vi "Process Array Elements.vi"(7 "Format String (%#0.15f)":string="%#0.15f", 8 "Error In":errorcluster, 9 "Name In":string, 10 "Array Variant":variant, 11 "Queue In":refnum<queue>) -> (0 "Error Out":errorcluster, 1 "Data Out":string, 3 "Queue Out":refnum<queue>)   [LabVIEW 2020]
doc: "This VI was created for use with the Read/Write Cluster VIs. It converts array elements of the cluster to strings to be written to file.\n\nFreeware from Moore Good Ideas, www.mooregoodideas.com. Do not remove this line."
uses:
  <vilib>/Utility/Data Type/NI_Data Type.lvlib
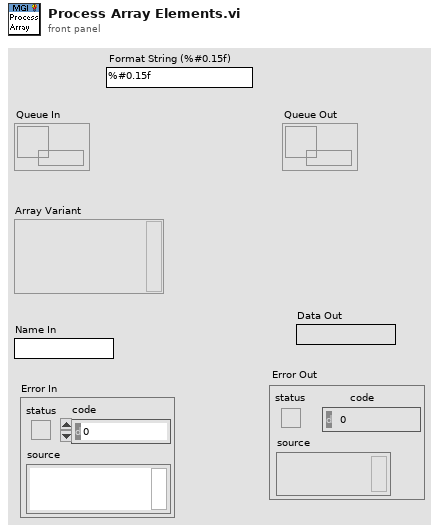
[diagram p1: front panel]
types:
  T1 = typedef "NI_Data Type.lvlib/Data Type.ctl" = enum8{"Invalid Type", "Void", "I8", "I16", "I32", "I64", "U8", "U16", "U32", "U64", "Single Float", "Double Float", "Extended Float", "Single Complex", "Double Complex", "Extended Complex", "Enum U8", "Enum U16", "Enum U32", "Enum U64", "Single Float With Unit", "Double Float With Unit", "Extended Float With Unit", "Single Complex with Unit", "Double Complex with Unit", "Extended Complex with Unit", "Boolean", "String", "Path", "Picture", "Tag", "Array", "Cluster", "Variant", "LV Variant", "Waveform", "Timestamp", "Digital Waveform", "Digital Data", "ExpressData", "Refnum", "External Data", "VI", "Poly VI", "LabVIEW Class Instance", "Fixed Point", "Set Collection", "Map Collection"}
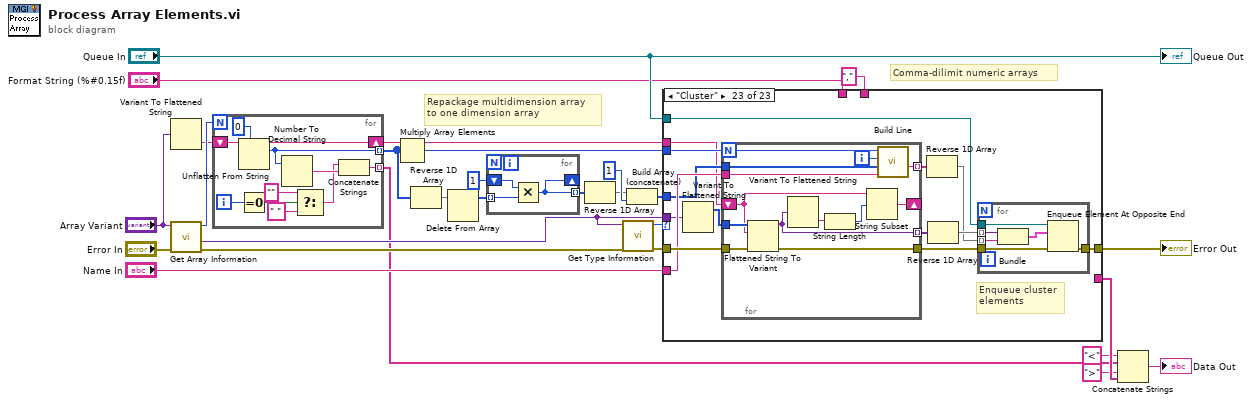
[diagram p0: block diagram]
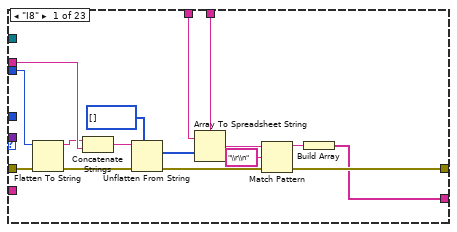
[diagram p2: hidden frame]
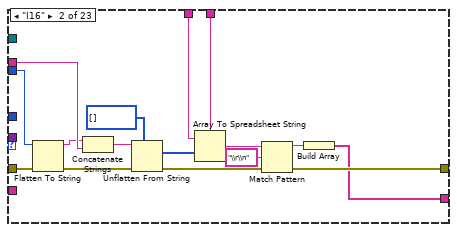
[diagram p3: hidden frame]
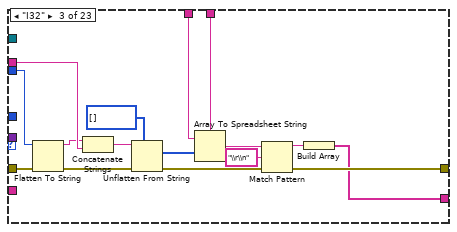
[diagram p4: hidden frame]
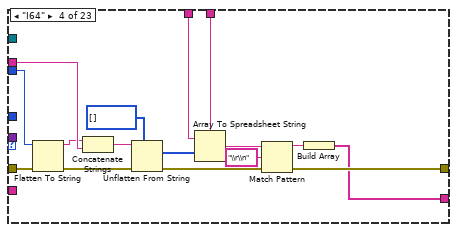
[diagram p5: hidden frame]
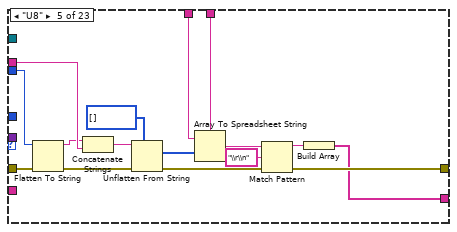
[diagram p6: hidden frame]
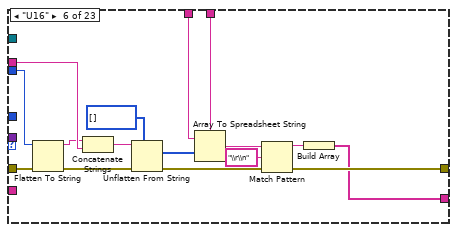
[diagram p7: hidden frame]
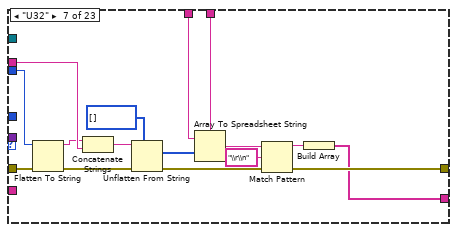
[diagram p8: hidden frame]
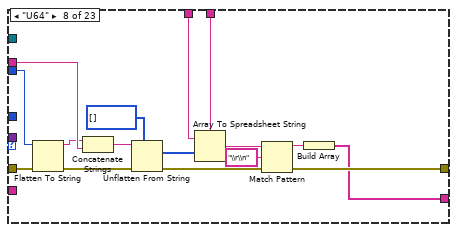
[diagram p9: hidden frame]
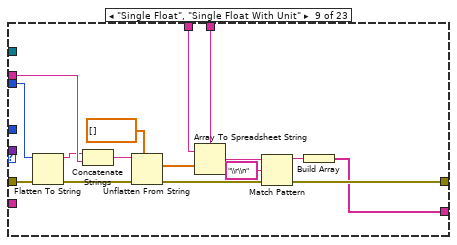
[diagram p10: hidden frame]
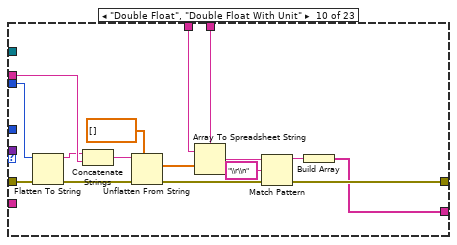
[diagram p11: hidden frame]
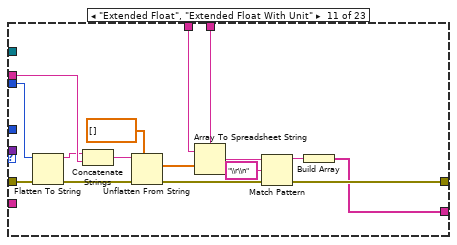
[diagram p12: hidden frame]
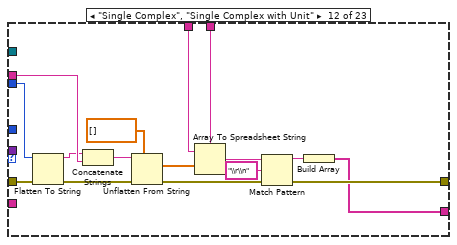
[diagram p13: hidden frame]
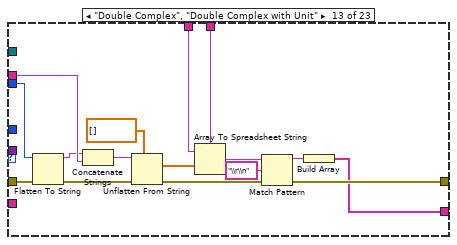
[diagram p14: hidden frame]
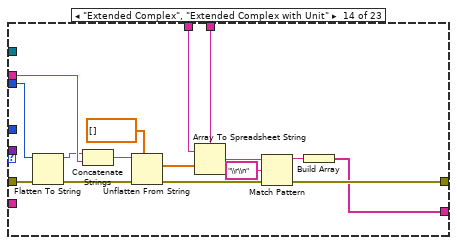
[diagram p15: hidden frame]
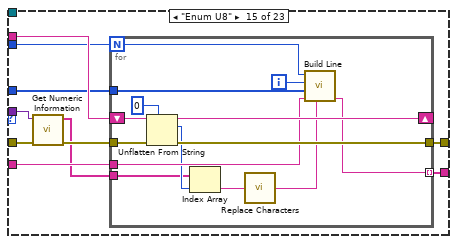
[diagram p16: hidden frame]
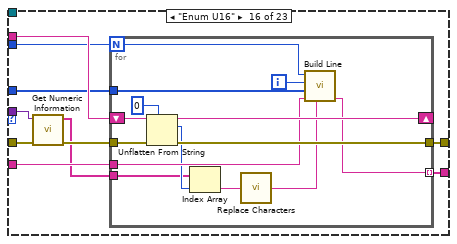
[diagram p17: hidden frame]
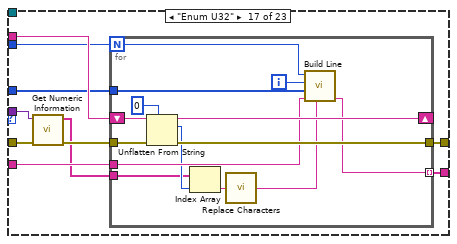
[diagram p18: hidden frame]
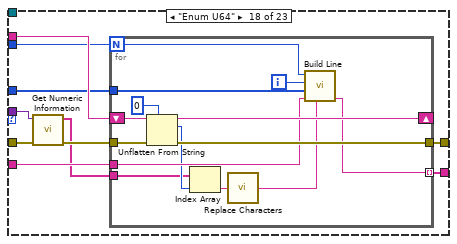
[diagram p19: hidden frame]
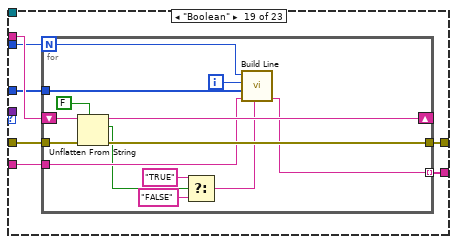
[diagram p20: hidden frame]
diagram:
  # "Comma-dilimit numeric arrays"
  # "Repackage multidimension array\nto one dimension array"
  n1 = Variant To Flattened String(Variant="Array Variant") -> (data string=w25:string)  [unwired: 1 out]
  n2 = call <vilib>:"Get Array Information.vi"("error in (no error)"="Error In", "variant"="Array Variant") -> ("error out"=w7:errorcluster, "array element data type"=w8:variant, "number of dimensions"=w26:i32)  [unwired: 6 in, 1 out]
  n3 = for {
    N: w26 -> [_]
    shift-right: [w37] -> w23
    shift-left: w25 -> [w38]
    tunnel: [w34] -> w12 mode=indexing
    tunnel: [w35] -> w6 mode=indexing
    i -> [w33]
    n4 = Unflatten From String(type=u32 0, binary string=w38) -> (rest of the binary string=w37:string, value=w34:u32)  [unwired: 3 in, 1 out]
    n5 = Equal To 0?(x=w33) -> (x = 0?=w32:bool)
    n6 = Number To Decimal String(number=w34) -> (decimal integer string=w36:string)  [unwired: 1 in]
    n7 = Select(t="", s=w32, f=" ") -> (s? t:f=w30:string)
    n8 = Concatenate Strings(w30, w36) -> (w35:string)
  }
  n9 = Multiply Array Elements(1:w12) -> (0:w22:u32)
  n10 = Reverse 1D Array(array=w12) -> (reversed array=w13:u32[])
  n11 = Delete From Array(array=w13) -> (array with subset deleted=w14:u32[])  [unwired: 2 in, 1 out]
  n12 = for {
    tunnel: w14 -> [w42] mode=indexing
    shift-right: [w40] -> _
    shift-left: i8 1 -> [w41]
    tunnel: [w40] -> w16 mode=indexing
    n13 = Multiply(x=w41, y=w42) -> (x*y=w40:u32)
  }
  n14 = Reverse 1D Array(array=w16) -> (reversed array=w17:u32[])
  n15 = call <vilib>:"Get Type Information.vi"("error in (no error)"=w7, "variant"=w8) -> ("error out"=w24:errorcluster, "type"=w3:T1)  [unwired: 5 in, 3 out]
  n16 = Build Array (concatenate)(w17, i8 1) -> (w11:u32[])
  n17 = case shown="\"Cluster\"" w3 {
    tunnel: [w57 w72 w87 w102 w117 w132 w147 w162 w177 w192 w207 w222 w237 w252 w262 w286 w310 w334 w355 w376 w395 w411 w421] -> w10
    tunnel: w24 -> [w46 w61 w76 w91 w106 w121 w136 w151 w166 w181 w196 w211 w226 w241 w255 w279 w303 w327 w354 w375 w394 w411 w429]
    tunnel: w23 -> [w56 w71 w86 w101 w116 w131 w146 w161 w176 w191 w206 w221 w236 w251 w261 w285 w309 w333 w353 w374 w393 w410 w416]
    tunnel: w22 -> [w55 w70 w85 w100 w115 w130 w145 w160 w175 w190 w205 w220 w235 w250 w260 w284 w308 w332 w352 w373 w392 _ w428]
    tunnel: "Name In" -> [_ _ _ _ _ _ _ _ _ _ _ _ _ _ w259 w283 w307 w331 w351 w372 w391 _ w427]
    tunnel: [w54 w69 w84 w99 w114 w129 w144 w159 w174 w189 w204 w219 w234 w249 w257 w281 w305 w329 w349 w370 w389 w409 _] -> w20
    tunnel: w11 -> [_ _ _ _ _ _ _ _ _ _ _ _ _ _ w258 w282 w306 w330 w350 w371 w390 _ w426]
    tunnel: "Queue In" -> [_ _ _ _ _ _ _ _ _ _ _ _ _ _ _ _ _ _ _ _ _ _ w422]
    tunnel: w8 -> [_ _ _ _ _ _ _ _ _ _ _ _ _ _ w256 w280 w304 w328 _ _ _ _ w419]
    tunnel: "Format String (%#0.15f)" -> [w44 w59 w74 w89 w104 w119 w134 w149 w164 w179 w194 w209 w224 w239 _ _ _ _ _ _ _ _ _]
    tunnel: "," ("delimiter (Tab)") -> [w43 w58 w73 w88 w103 w118 w133 w148 w163 w178 w193 w208 w223 w238 _ _ _ _ _ _ _ _ _]
    frame "I8" {
      n18 = Flatten To String(anything=w55, error in (no error)=w46) -> (data string=w51:string, error out=w45:errorcluster)  [unwired: 2 in, 1 out]
      n19 = Concatenate Strings(w51, w56) -> (w52:string)
      n20 = Unflatten From String(type=i8[] [], binary string=w52, error in (no error)=w45) -> (value=w48:i8[], error out=w57:errorcluster)  [unwired: 2 in, 1 out]
      n21 = Array To Spreadsheet String(delimiter (Tab)=w43, array=w48, 3:w44) -> (spreadsheet string=w50:string)
      n22 = Match Pattern(string=w50, regular expression="\\r\\n") -> (before substring=w47:string)  [unwired: 1 in, 3 out]
      n23 = Build Array(w47) -> (w54:string[])
    }
    frame "I16" {
      n24 = Flatten To String(anything=w70, error in (no error)=w61) -> (data string=w66:string, error out=w60:errorcluster)  [unwired: 2 in, 1 out]
      n25 = Concatenate Strings(w66, w71) -> (w67:string)
      n26 = Unflatten From String(type=i16[] [], binary string=w67, error in (no error)=w60) -> (value=w63:i16[], error out=w72:errorcluster)  [unwired: 2 in, 1 out]
      n27 = Array To Spreadsheet String(delimiter (Tab)=w58, array=w63, 3:w59) -> (spreadsheet string=w65:string)
      n28 = Match Pattern(string=w65, regular expression="\\r\\n") -> (before substring=w62:string)  [unwired: 1 in, 3 out]
      n29 = Build Array(w62) -> (w69:string[])
    }
    frame "I32" {
      n30 = Flatten To String(anything=w85, error in (no error)=w76) -> (data string=w81:string, error out=w75:errorcluster)  [unwired: 2 in, 1 out]
      n31 = Concatenate Strings(w81, w86) -> (w82:string)
      n32 = Unflatten From String(type=i32[] [], binary string=w82, error in (no error)=w75) -> (value=w78:i32[], error out=w87:errorcluster)  [unwired: 2 in, 1 out]
      n33 = Array To Spreadsheet String(delimiter (Tab)=w73, array=w78, 3:w74) -> (spreadsheet string=w80:string)
      n34 = Match Pattern(string=w80, regular expression="\\r\\n") -> (before substring=w77:string)  [unwired: 1 in, 3 out]
      n35 = Build Array(w77) -> (w84:string[])
    }
    frame "I64" {
      n36 = Flatten To String(anything=w100, error in (no error)=w91) -> (data string=w96:string, error out=w90:errorcluster)  [unwired: 2 in, 1 out]
      n37 = Concatenate Strings(w96, w101) -> (w97:string)
      n38 = Unflatten From String(type=i64[] [], binary string=w97, error in (no error)=w90) -> (value=w93:i64[], error out=w102:errorcluster)  [unwired: 2 in, 1 out]
      n39 = Array To Spreadsheet String(delimiter (Tab)=w88, array=w93, 3:w89) -> (spreadsheet string=w95:string)
      n40 = Match Pattern(string=w95, regular expression="\\r\\n") -> (before substring=w92:string)  [unwired: 1 in, 3 out]
      n41 = Build Array(w92) -> (w99:string[])
    }
    frame "U8" {
      n42 = Flatten To String(anything=w115, error in (no error)=w106) -> (data string=w111:string, error out=w105:errorcluster)  [unwired: 2 in, 1 out]
      n43 = Concatenate Strings(w111, w116) -> (w112:string)
      n44 = Unflatten From String(type=u8[] [], binary string=w112, error in (no error)=w105) -> (value=w108:u8[], error out=w117:errorcluster)  [unwired: 2 in, 1 out]
      n45 = Array To Spreadsheet String(delimiter (Tab)=w103, array=w108, 3:w104) -> (spreadsheet string=w110:string)
      n46 = Match Pattern(string=w110, regular expression="\\r\\n") -> (before substring=w107:string)  [unwired: 1 in, 3 out]
      n47 = Build Array(w107) -> (w114:string[])
    }
    frame "U16" {
      n48 = Flatten To String(anything=w130, error in (no error)=w121) -> (data string=w126:string, error out=w120:errorcluster)  [unwired: 2 in, 1 out]
      n49 = Concatenate Strings(w126, w131) -> (w127:string)
      n50 = Unflatten From String(type=u16[] [], binary string=w127, error in (no error)=w120) -> (value=w123:u16[], error out=w132:errorcluster)  [unwired: 2 in, 1 out]
      n51 = Array To Spreadsheet String(delimiter (Tab)=w118, array=w123, 3:w119) -> (spreadsheet string=w125:string)
      n52 = Match Pattern(string=w125, regular expression="\\r\\n") -> (before substring=w122:string)  [unwired: 1 in, 3 out]
      n53 = Build Array(w122) -> (w129:string[])
    }
    frame "U32" {
      n54 = Flatten To String(anything=w145, error in (no error)=w136) -> (data string=w141:string, error out=w135:errorcluster)  [unwired: 2 in, 1 out]
      n55 = Concatenate Strings(w141, w146) -> (w142:string)
      n56 = Unflatten From String(type=u32[] [], binary string=w142, error in (no error)=w135) -> (value=w138:u32[], error out=w147:errorcluster)  [unwired: 2 in, 1 out]
      n57 = Array To Spreadsheet String(delimiter (Tab)=w133, array=w138, 3:w134) -> (spreadsheet string=w140:string)
      n58 = Match Pattern(string=w140, regular expression="\\r\\n") -> (before substring=w137:string)  [unwired: 1 in, 3 out]
      n59 = Build Array(w137) -> (w144:string[])
    }
    frame "U64" {
      n60 = Flatten To String(anything=w160, error in (no error)=w151) -> (data string=w156:string, error out=w150:errorcluster)  [unwired: 2 in, 1 out]
      n61 = Concatenate Strings(w156, w161) -> (w157:string)
      n62 = Unflatten From String(type=u64[] [], binary string=w157, error in (no error)=w150) -> (value=w153:u64[], error out=w162:errorcluster)  [unwired: 2 in, 1 out]
      n63 = Array To Spreadsheet String(delimiter (Tab)=w148, array=w153, 3:w149) -> (spreadsheet string=w155:string)
      n64 = Match Pattern(string=w155, regular expression="\\r\\n") -> (before substring=w152:string)  [unwired: 1 in, 3 out]
      n65 = Build Array(w152) -> (w159:string[])
    }
    frame "Single Float", "Single Float With Unit" {
      n66 = Flatten To String(anything=w175, error in (no error)=w166) -> (data string=w171:string, error out=w165:errorcluster)  [unwired: 2 in, 1 out]
      n67 = Concatenate Strings(w171, w176) -> (w172:string)
      n68 = Unflatten From String(type=sgl[] [], binary string=w172, error in (no error)=w165) -> (value=w168:sgl[], error out=w177:errorcluster)  [unwired: 2 in, 1 out]
      n69 = Array To Spreadsheet String(delimiter (Tab)=w163, array=w168, 3:w164) -> (spreadsheet string=w170:string)
      n70 = Match Pattern(string=w170, regular expression="\\r\\n") -> (before substring=w167:string)  [unwired: 1 in, 3 out]
      n71 = Build Array(w167) -> (w174:string[])
    }
    frame "Double Float", "Double Float With Unit" {
      n72 = Flatten To String(anything=w190, error in (no error)=w181) -> (data string=w186:string, error out=w180:errorcluster)  [unwired: 2 in, 1 out]
      n73 = Concatenate Strings(w186, w191) -> (w187:string)
      n74 = Unflatten From String(type=dbl[] [], binary string=w187, error in (no error)=w180) -> (value=w183:dbl[], error out=w192:errorcluster)  [unwired: 2 in, 1 out]
      n75 = Array To Spreadsheet String(delimiter (Tab)=w178, array=w183, 3:w179) -> (spreadsheet string=w185:string)
      n76 = Match Pattern(string=w185, regular expression="\\r\\n") -> (before substring=w182:string)  [unwired: 1 in, 3 out]
      n77 = Build Array(w182) -> (w189:string[])
    }
    frame "Extended Float", "Extended Float With Unit" {
      n78 = Flatten To String(anything=w205, error in (no error)=w196) -> (data string=w201:string, error out=w195:errorcluster)  [unwired: 2 in, 1 out]
      n79 = Concatenate Strings(w201, w206) -> (w202:string)
      n80 = Unflatten From String(type=ext[] [], binary string=w202, error in (no error)=w195) -> (value=w198:ext[], error out=w207:errorcluster)  [unwired: 2 in, 1 out]
      n81 = Array To Spreadsheet String(delimiter (Tab)=w193, array=w198, 3:w194) -> (spreadsheet string=w200:string)
      n82 = Match Pattern(string=w200, regular expression="\\r\\n") -> (before substring=w197:string)  [unwired: 1 in, 3 out]
      n83 = Build Array(w197) -> (w204:string[])
    }
    frame "Single Complex", "Single Complex with Unit" {
      n84 = Flatten To String(anything=w220, error in (no error)=w211) -> (data string=w216:string, error out=w210:errorcluster)  [unwired: 2 in, 1 out]
      n85 = Concatenate Strings(w216, w221) -> (w217:string)
      n86 = Unflatten From String(type=csg[] [], binary string=w217, error in (no error)=w210) -> (value=w213:csg[], error out=w222:errorcluster)  [unwired: 2 in, 1 out]
      n87 = Array To Spreadsheet String(delimiter (Tab)=w208, array=w213, 3:w209) -> (spreadsheet string=w215:string)
      n88 = Match Pattern(string=w215, regular expression="\\r\\n") -> (before substring=w212:string)  [unwired: 1 in, 3 out]
      n89 = Build Array(w212) -> (w219:string[])
    }
    frame "Double Complex", "Double Complex with Unit" {
      n90 = Flatten To String(anything=w235, error in (no error)=w226) -> (data string=w231:string, error out=w225:errorcluster)  [unwired: 2 in, 1 out]
      n91 = Concatenate Strings(w231, w236) -> (w232:string)
      n92 = Unflatten From String(type=cdb[] [], binary string=w232, error in (no error)=w225) -> (value=w228:cdb[], error out=w237:errorcluster)  [unwired: 2 in, 1 out]
      n93 = Array To Spreadsheet String(delimiter (Tab)=w223, array=w228, 3:w224) -> (spreadsheet string=w230:string)
      n94 = Match Pattern(string=w230, regular expression="\\r\\n") -> (before substring=w227:string)  [unwired: 1 in, 3 out]
      n95 = Build Array(w227) -> (w234:string[])
    }
    frame "Extended Complex", "Extended Complex with Unit" {
      n96 = Flatten To String(anything=w250, error in (no error)=w241) -> (data string=w246:string, error out=w240:errorcluster)  [unwired: 2 in, 1 out]
      n97 = Concatenate Strings(w246, w251) -> (w247:string)
      n98 = Unflatten From String(type=cxt[] [], binary string=w247, error in (no error)=w240) -> (value=w243:cxt[], error out=w252:errorcluster)  [unwired: 2 in, 1 out]
      n99 = Array To Spreadsheet String(delimiter (Tab)=w238, array=w243, 3:w239) -> (spreadsheet string=w245:string)
      n100 = Match Pattern(string=w245, regular expression="\\r\\n") -> (before substring=w242:string)  [unwired: 1 in, 3 out]
      n101 = Build Array(w242) -> (w249:string[])
    }
    frame "Enum U8" {
      n102 = call <vilib>:"Get Numeric Information.vi"("error in (no error)"=w255, "variant"=w256) -> ("error out"=w254:errorcluster, "enum names"=w253:string[])  [unwired: 6 in, 2 out]
      n103 = for {
        N: w260 -> [w272]
        tunnel: [w273] -> w262
        tunnel: w254 -> [w274]
        shift-right: [w275] -> _
        shift-left: w261 -> [w276]
        tunnel: w259 -> [w268]
        tunnel: [w269] -> w257 mode=indexing
        tunnel: w258 -> [w270]
        tunnel: w253 -> [w265]
        i -> [w271]
        n104 = Unflatten From String(type=u8 0, binary string=w276, error in (no error)=w274) -> (rest of the binary string=w275:string, value=w266:u8, error out=w273:errorcluster)  [unwired: 2 in]
        n105 = Index Array(array=w265, index=w266) -> (element=w264:string)
        n106 = call "Replace Characters.vi"("String In"=w264) -> ("String Out"=w263:string)  [unwired: 1 in]
        n107 = call "Build Line.vi"("Value String (\"\")"=w263, "Name In"=w268, "Array"=w270, "Iteration"=w271, "Iterations"=w272) -> ("Line"=w269:string)  [unwired: 5 in, 1 out]
      }
    }
    frame "Enum U16" {
      n108 = call <vilib>:"Get Numeric Information.vi"("error in (no error)"=w279, "variant"=w280) -> ("error out"=w278:errorcluster, "enum names"=w277:string[])  [unwired: 6 in, 2 out]
      n109 = for {
        N: w284 -> [w296]
        tunnel: [w297] -> w286
        tunnel: w278 -> [w298]
        shift-right: [w299] -> _
        shift-left: w285 -> [w300]
        tunnel: w283 -> [w292]
        tunnel: [w293] -> w281 mode=indexing
        tunnel: w282 -> [w294]
        tunnel: w277 -> [w289]
        i -> [w295]
        n110 = Unflatten From String(type=u16 0, binary string=w300, error in (no error)=w298) -> (rest of the binary string=w299:string, value=w290:u16, error out=w297:errorcluster)  [unwired: 2 in]
        n111 = Index Array(array=w289, index=w290) -> (element=w288:string)
        n112 = call "Replace Characters.vi"("String In"=w288) -> ("String Out"=w287:string)  [unwired: 1 in]
        n113 = call "Build Line.vi"("Value String (\"\")"=w287, "Name In"=w292, "Array"=w294, "Iteration"=w295, "Iterations"=w296) -> ("Line"=w293:string)  [unwired: 5 in, 1 out]
      }
    }
    frame "Enum U32" {
      n114 = call <vilib>:"Get Numeric Information.vi"("error in (no error)"=w303, "variant"=w304) -> ("error out"=w302:errorcluster, "enum names"=w301:string[])  [unwired: 6 in, 2 out]
      n115 = for {
        N: w308 -> [w320]
        tunnel: [w321] -> w310
        tunnel: w302 -> [w322]
        shift-right: [w323] -> _
        shift-left: w309 -> [w324]
        tunnel: w307 -> [w316]
        tunnel: [w317] -> w305 mode=indexing
        tunnel: w306 -> [w318]
        tunnel: w301 -> [w313]
        i -> [w319]
        n116 = Unflatten From String(type=u32 0, binary string=w324, error in (no error)=w322) -> (rest of the binary string=w323:string, value=w314:u32, error out=w321:errorcluster)  [unwired: 2 in]
        n117 = Index Array(array=w313, index=w314) -> (element=w312:string)
        n118 = call "Replace Characters.vi"("String In"=w312) -> ("String Out"=w311:string)  [unwired: 1 in]
        n119 = call "Build Line.vi"("Value String (\"\")"=w311, "Name In"=w316, "Array"=w318, "Iteration"=w319, "Iterations"=w320) -> ("Line"=w317:string)  [unwired: 5 in, 1 out]
      }
    }
    frame "Enum U64" {
      n120 = call <vilib>:"Get Numeric Information.vi"("error in (no error)"=w327, "variant"=w328) -> ("error out"=w326:errorcluster, "enum names"=w325:string[])  [unwired: 6 in, 2 out]
      n121 = for {
        N: w332 -> [w344]
        tunnel: [w345] -> w334
        tunnel: w326 -> [w346]
        shift-right: [w347] -> _
        shift-left: w333 -> [w348]
        tunnel: w331 -> [w340]
        tunnel: [w341] -> w329 mode=indexing
        tunnel: w330 -> [w342]
        tunnel: w325 -> [w337]
        i -> [w343]
        n122 = Unflatten From String(type=u64 0, binary string=w348, error in (no error)=w346) -> (rest of the binary string=w347:string, value=w338:u64, error out=w345:errorcluster)  [unwired: 2 in]
        n123 = Index Array(array=w337, index=w338) -> (element=w336:string)
        n124 = call "Replace Characters.vi"("String In"=w336) -> ("String Out"=w335:string)  [unwired: 1 in]
        n125 = call "Build Line.vi"("Value String (\"\")"=w335, "Name In"=w340, "Array"=w342, "Iteration"=w343, "Iterations"=w344) -> ("Line"=w341:string)  [unwired: 5 in, 1 out]
      }
    }
    frame "Boolean" {
      n126 = for {
        N: w352 -> [w365]
        tunnel: [w366] -> w355
        tunnel: w354 -> [w367]
        shift-right: [w368] -> _
        shift-left: w353 -> [w369]
        tunnel: w351 -> [w361]
        tunnel: [w362] -> w349 mode=indexing
        tunnel: w350 -> [w363]
        i -> [w364]
        n127 = Unflatten From String(type=FALSE, binary string=w369, error in (no error)=w367) -> (rest of the binary string=w368:string, value=w357:bool, error out=w366:errorcluster)  [unwired: 2 in]
        n128 = Select(t="TRUE", s=w357, f="FALSE") -> (s? t:f=w356:string)
        n129 = call "Build Line.vi"("Value String (\"\")"=w356, "Name In"=w361, "Array"=w363, "Iteration"=w364, "Iterations"=w365) -> ("Line"=w362:string)  [unwired: 5 in, 1 out]
      }
    }
    frame "String" {
      n130 = for {
        N: w373 -> [w384]
        tunnel: [w385] -> w376
        tunnel: w375 -> [w386]
        shift-right: [w387] -> _
        shift-left: w374 -> [w388]
        tunnel: w372 -> [w380]
        tunnel: [w381] -> w370 mode=indexing
        tunnel: w371 -> [w382]
        i -> [w383]
        n131 = Unflatten From String(type="", binary string=w388, error in (no error)=w386) -> (rest of the binary string=w387:string, value=w378:string, error out=w385:errorcluster)  [unwired: 2 in]
        n132 = call "Replace Characters.vi"("String In"=w378) -> ("String Out"=w377:string)  [unwired: 1 in]
        n133 = call "Build Line.vi"("Value String (\"\")"=w377, "Name In"=w380, "Array"=w382, "Iteration"=w383, "Iterations"=w384) -> ("Line"=w381:string)  [unwired: 5 in, 1 out]
      }
    }
    frame "Path" {
      n134 = for {
        N: w392 -> [w404]
        tunnel: [w405] -> w395
        tunnel: w394 -> [w406]
        shift-right: [w407] -> _
        shift-left: w393 -> [w408]
        tunnel: w391 -> [w400]
        tunnel: [w401] -> w389 mode=indexing
        tunnel: w390 -> [w402]
        i -> [w403]
        n135 = Unflatten From String(type=path "", binary string=w408, error in (no error)=w406) -> (rest of the binary string=w407:string, value=w398:path, error out=w405:errorcluster)  [unwired: 2 in]
        n136 = Path To String(path=w398) -> (string=w397:string)
        n137 = call "Replace Characters.vi"("String In"=w397) -> ("String Out"=w396:string)  [unwired: 1 in]
        n138 = call "Build Line.vi"("Value String (\"\")"=w396, "Name In"=w400, "Array"=w402, "Iteration"=w403, "Iterations"=w404) -> ("Line"=w401:string)  [unwired: 5 in, 1 out]
      }
    }
    frame Default {
      n139 = String To Byte Array(string=w410) -> (unsigned byte array=w415:u8[])
      n140 = Number To Hexadecimal String(1:i16 2 ("width (-)"), 2:w415) -> (0:w414:string[])
      n141 = Build Array (concatenate)("0x", w414) -> (w409:string[])
    }
    frame "Cluster" {
      # "Enqueue cluster\nelements"
      n142 = Variant To Flattened String(Variant=w419) -> (1:w418:i16[])  [unwired: 1 out]
      n143 = for {
        N: w428 -> [w448]
        tunnel: [w442] -> w423
        tunnel: w429 -> [w444]
        tunnel: w427 -> [w439]
        tunnel: w426 -> [w446]
        tunnel: [w440] -> w424 mode=indexing
        tunnel: [w445] -> w420 mode=indexing
        tunnel: w418 -> [w443]
        shift-right: [w436] -> _
        shift-left: w416 -> [w437]
        i -> [w447]
        n144 = Flattened String To Variant(4:w444, 6:w437, 7:w443) -> (0:w442:errorcluster, 3:w440:variant)
        n145 = Variant To Flattened String(Variant=w440) -> (data string=w441:string)  [unwired: 1 out]
        n146 = String Length(string=w441) -> (length=w438:i32)
        n147 = String Subset(string=w437, offset (0)=w438) -> (substring=w436:string)  [unwired: 1 in]
        n148 = call "Build Line.vi"("Name In"=w439, "Array"=w446, "Iteration"=w447, "Iterations"=w448) -> ("Name Out"=w445:string)  [unwired: 6 in, 1 out]
      }
      n149 = Reverse 1D Array(array=w420) -> (reversed array=w417:string[])
      n150 = Reverse 1D Array(array=w424) -> (reversed array=w425:variant[])
      n151 = for {
        tunnel: [w435] -> w421
        tunnel: w425 -> [w434] mode=indexing
        tunnel: w423 -> [w433]
        tunnel: w422 -> [w431]
        tunnel: w417 -> [w430] mode=indexing
        n152 = Bundle("Variant"=w434, "Name Out"=w430) -> (w432:cluster{"Variant":variant, "Name Out":string})  [unwired: 1 in]
        n153 = Enqueue Element At Opposite End(queue=w431, element=w432, error in (no error)=w433) -> (error out=w435:errorcluster)  [unwired: 1 in, 2 out]
      }
    }
  }
  "Error Out" <- w10
  n154 = Concatenate Strings("<", w6, ">", w20) -> (→"Data Out":string)
  "Queue Out" <- "Queue In"
